vi "String2CharArray.vi"(4 "String In":string) -> (1 "Char Array":string[](array[string]))   [LabVIEW 2020]
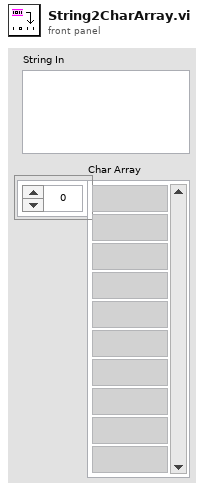
[diagram p1: front panel]
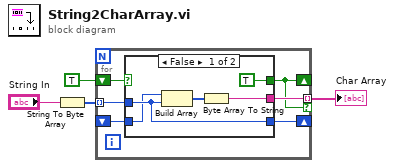
[diagram p0: block diagram]
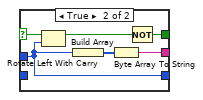
[diagram p2: hidden frame]
diagram:
  n1 = String To Byte Array(string="String In") -> (unsigned byte array=w2:u8[])
  n2 = for {
    tunnel: w2 -> [w10] mode=indexing
    shift-right: [w7] -> _
    shift-left: TRUE -> [w9]
    tunnel: [w8] -> w3 mode=indexing if=w7
    shift-right: [w5] -> _
    shift-left: _ -> [w6]
    n3 = case shown="False" w9 {
      selector: w9 -> [_ w16]
      tunnel: w10 -> [w14 w17]
      tunnel: [TRUE w20] -> w7
      tunnel: [w11 w18] -> w8
      tunnel: [w14 w17] -> w5
      tunnel: w6 -> [w13 _]
      frame False {
        n4 = Build Array(w13, w14) -> (w12:u8[])
        n5 = Byte Array To String(unsigned byte array=w12) -> (string=w11:string)
      }
      frame True {
        n6 = Rotate Left With Carry(2:w17, 3:w16) -> (1:w21:bool)  [unwired: 1 out]
        n7 = Build Array(w17) -> (w19:u8[])
        n8 = Byte Array To String(unsigned byte array=w19) -> (string=w18:string)
        n9 = Not(x=w21) -> (.not. x?=w20:bool)
      }
    }
  }
  "Char Array" <- w3
